vi "InitState.vi"(0 "Error In":errorcluster, 3 "Name":string) -> (7 "Error Out":errorcluster, 10 "Queue Out":refnum<queue>)   [LabVIEW 2010]
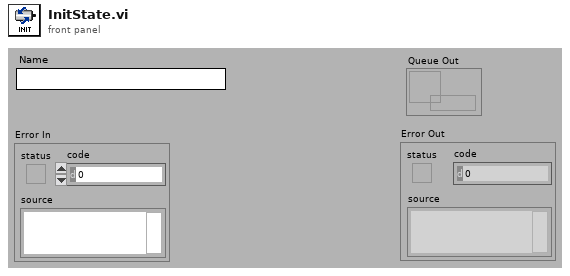
[diagram p1: front panel]
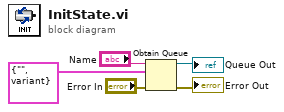
[diagram p0: block diagram]
diagram:
  n1 = Obtain Queue(name (unnamed)="Name", element data type=cluster{"State":string, "Data":variant} {"State"="", "Data"=variant}, error in (no error)="Error In") -> (queue out=→"Queue Out":refnum<queue>, error out=→"Error Out":errorcluster)  [unwired: 2 in, 1 out]
